vi "Init Msg Output.vi"() -> (2 "Msg Output":refnum<class "Msg Output.lvclass">)   [LabVIEW 2025, in "_Template.lvlib" / "Templates.lvlib" / "TEMPLATE jettl Msg.lvlib" / "TEMPLATE Msg Output.lvlib"]
uses:
  TEMPLATE Msg Output.lvlib
  jettl/jettl/Msg Output/Msg Output.lvclass
  TEMPLATE Msg Output/TEMPLATE Msg Output.lvclass
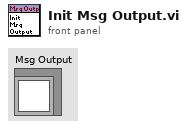
[diagram p1: front panel]
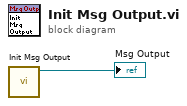
[diagram p0: block diagram]
diagram:
  n1 = call "Init Msg Output.vi"() -> ("TEMPLATE Msg Output out"=→"Msg Output":refnum<class "TEMPLATE Msg Output.lvclass">)  [unwired: 11 in]
